vi "BlackJack.vi"() -> ()   [LabVIEW 2018]
panel:
  in  "Description":bool
  in  "Deal cards":bool
  in  "End the game":bool
  out "Dealer's Card":u16[](array[ring])
  out "Your Card":u16[](array[ring])
  out "Result":string
  in  "Number of decks":i32=1
  in  "Chips in hand":dbl=10.0
  in  "Bet":dbl=1.0
  in  "Blackjack odds":dbl=1.5
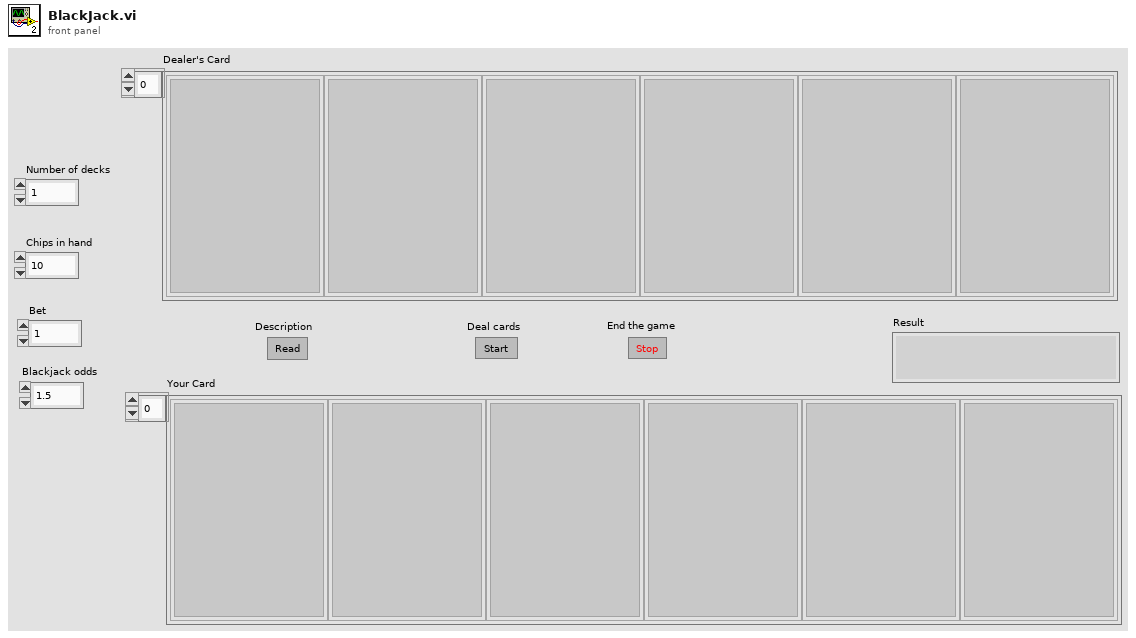
[diagram p1: front panel]
types:
  T1 = enum16{"Left Button", "Center Button", "Right Button", "Window Close"}
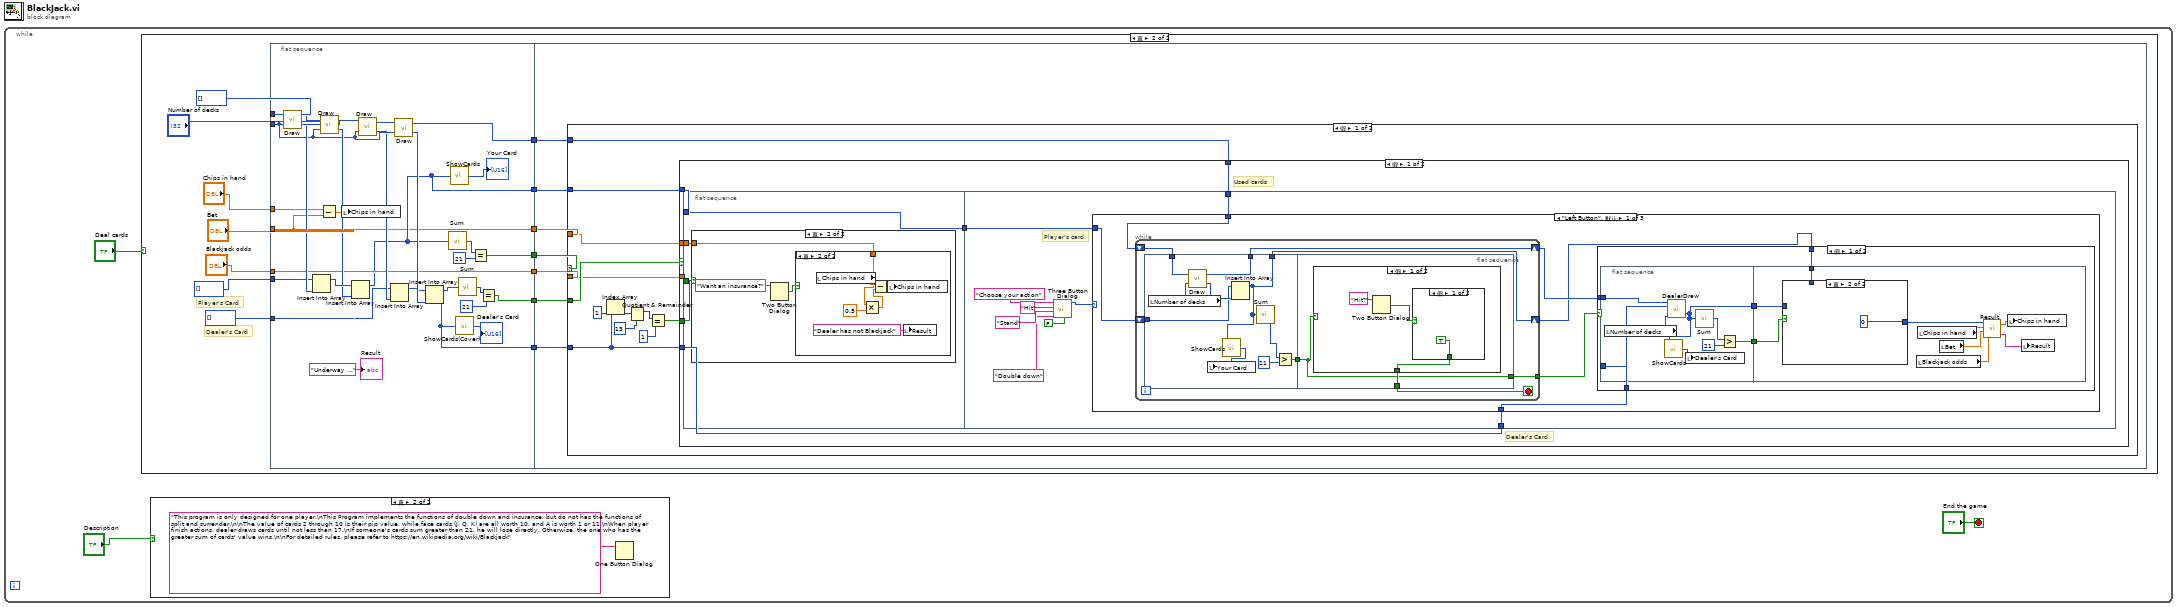
[diagram p0: block diagram]
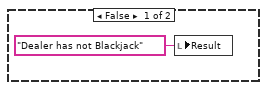
[diagram p5: hidden frame]
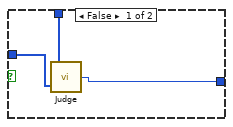
[diagram p6: hidden frame]
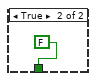
[diagram p8: hidden frame]
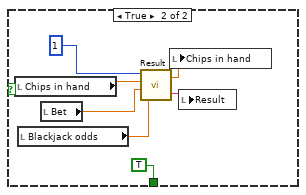
[diagram p9: hidden frame]
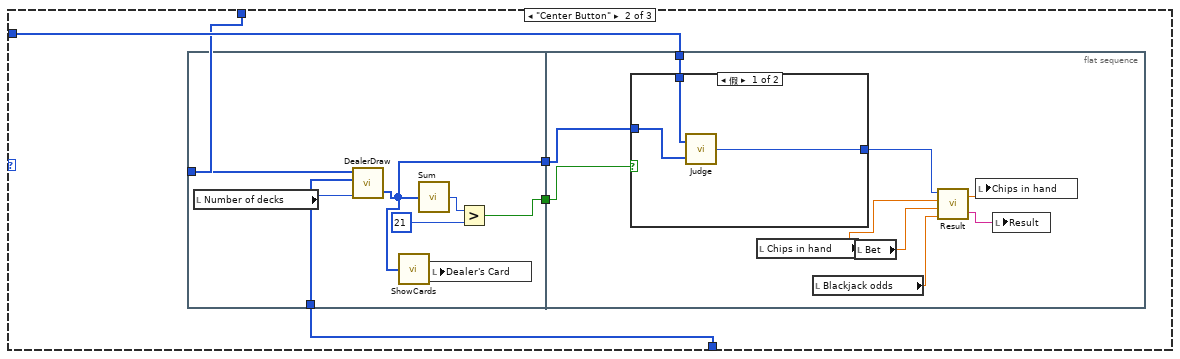
[diagram p10: hidden frame]
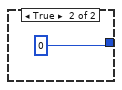
[diagram p11: hidden frame]
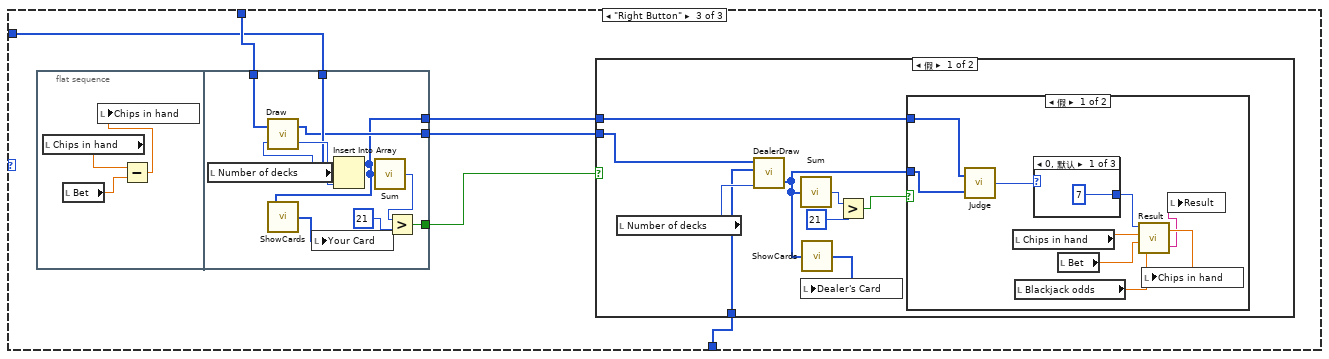
[diagram p12: hidden frame]
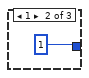
[diagram p13: hidden frame]
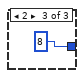
[diagram p14: hidden frame]
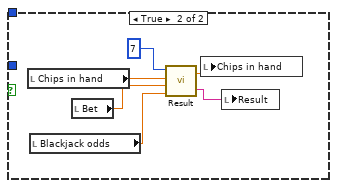
[diagram p15: hidden frame]
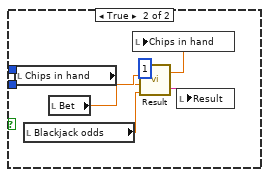
[diagram p16: hidden frame]
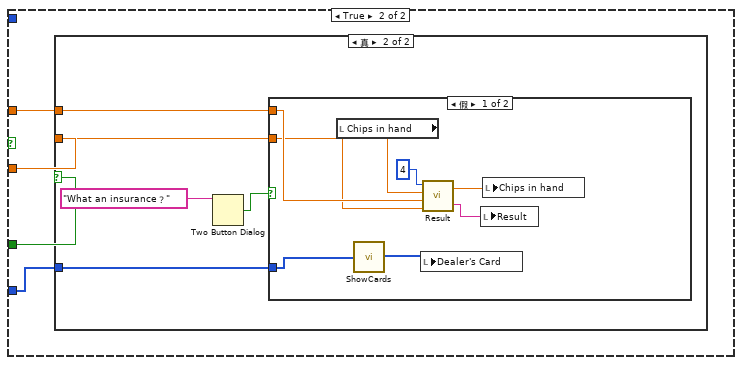
[diagram p17: hidden frame]
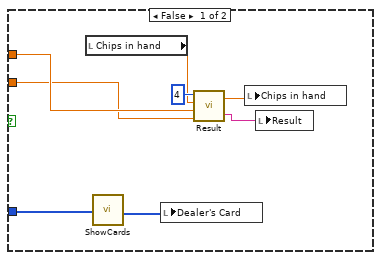
[diagram p18: hidden frame]
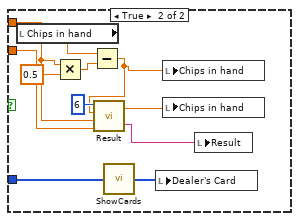
[diagram p19: hidden frame]
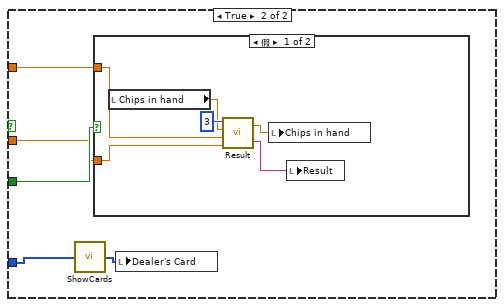
[diagram p20: hidden frame]
diagram:
  n1 = while {
    stop <- "End the game" stop-if-true
    n2 = case shown="真" "Deal cards" {
      frame False {
      }
      frame True {
        # "Player's Card"
        # "Dealer's Card"
        n3 = flat-sequence {
          tunnel: i32[] [] ("输入已用牌") -> [w47]
          tunnel: "Number of decks" -> [w39]
          tunnel: i32[] [] ("数组") -> [w45]
          tunnel: i32[] [] ("数组") -> [w36]
          tunnel: "Bet" -> [w21]
          tunnel: "Blackjack odds" -> [w29]
          tunnel: [w21] -> w18
          tunnel: [w29] -> w17
          tunnel: [w28] -> w16
          tunnel: [w27] -> w15
          tunnel: [w26] -> w14
          tunnel: [w25] -> w13
          tunnel: [w24] -> w12
          tunnel: "Chips in hand" -> [w20]
          tunnel: w18 -> [w54]
          tunnel: w17 -> [w53]
          tunnel: w16 -> [w52]
          tunnel: w15 -> [w51]
          tunnel: w14 -> [w50]
          tunnel: w13 -> [w49]
          tunnel: w12 -> [w48]
          frame #0 {
            n4 = call "Draw.vi"("Number of decks"=w39, "Input used cards"=w47) -> ("No. of card"=w46:i32, "Output used cards"=w44:i32[])
            n5 = Insert Into Array(array=w45, new element=w46) -> (w43:i32[])  [unwired: 1 in]
            n6 = call "Draw.vi"("Number of decks"=w39, "Input used cards"=w44) -> ("No. of card"=w42:i32, "Output used cards"=w41:i32[])
            n7 = Subtract(x=w20, y=w21) -> (x-y=w19:dbl)
            n8 = local write "Chips in hand"(w19) -> ()
            n9 = Insert Into Array(array=w43, new element=w42) -> (w24:i32[])  [unwired: 1 in]
            n10 = call "Draw.vi"("Number of decks"=w39, "Input used cards"=w41) -> ("No. of card"=w38:i32, "Output used cards"=w40:i32[])
            n11 = Insert Into Array(array=w36, new element=w38) -> (w35:i32[])  [unwired: 1 in]
            n12 = call "Draw.vi"("Number of decks"=w39, "Input used cards"=w40) -> ("No. of card"=w37:i32, "Output used cards"=w25:i32[])
            n13 = Insert Into Array(array=w35, new element=w37) -> (w26:i32[])  [unwired: 1 in]
            n14 = call "Sum.vi"("Array"=w24) -> ("Value"=w34:i32)
            n15 = call "ShowCards.vi"("Array 2"=w24) -> ("Array"=→"Your Card":u16[])
            n16 = call "ShowCards(Cover).vi"("Array"=w26) -> ("Array 2"=→"Dealer's Card":u16[])
            n17 = call "Sum.vi"("Array"=w26) -> ("Value"=w32:i32)
            n18 = Equal?(x=w34, y=21) -> (x = y?=w28:bool)
            n19 = Equal?(x=w32, y=21) -> (x = y?=w27:bool)
            "Result" <- "Underway ..." ("结果")
          }
          frame #1 {
            n20 = case shown="假" w52 {
              tunnel: w51 -> [w61 w276]
              tunnel: w54 -> [w59 w275]
              tunnel: w53 -> [w58 w274]
              tunnel: w50 -> [w66 w273]
              tunnel: w49 -> [w57 _]
              tunnel: w48 -> [w56 _]
              frame False {
                n21 = Index Array(array=w66, index=1 ("索引")) -> (element=w65:i32)
                n22 = Quotient & Remainder(x=w65, y=13) -> (x-y*floor(x/y)=w55:i32)  [unwired: 1 out]
                n23 = Equal?(x=w55, y=1) -> (x = y?=w60:bool)
                n24 = case shown="假" w61 {
                  tunnel: w66 -> [w67 w236]
                  tunnel: w60 -> [w72 w239]
                  tunnel: w59 -> [w71 w238]
                  tunnel: w58 -> [_ w237]
                  tunnel: w57 -> [w70 _]
                  tunnel: w56 -> [w68 _]
                  frame False {
                    # "Dealer's Card"
                    # "Used cards"
                    n25 = flat-sequence {
                      tunnel: w72 -> [w75]
                      tunnel: w71 -> [w74]
                      tunnel: [w73] -> w69
                      tunnel: w68 -> [w73]
                      tunnel: w70 -> [w88]
                      tunnel: w69 -> [w87]
                      tunnel: w67 -> [w86]
                      frame #0 {
                        n26 = case shown="真" w75 {
                          tunnel: w74 -> [_ w76]
                          frame False {
                          }
                          frame True {
                            n27 = Two Button Dialog(message="Want an insurance?" ("消息")) -> (T button?=w77:bool)  [unwired: 2 in]
                            n28 = case shown="真" w77 {
                              tunnel: w76 -> [_ w83]
                              frame False {
                                n29 = local write "Result"("Dealer has not Blackjack" ("结果")) -> ()
                              }
                              frame True {
                                n30 = local read "Chips in hand"() -> (w85:dbl)
                                n31 = Multiply(x=w83, y=0.5) -> (x*y=w81:dbl)
                                n32 = Subtract(x=w85, y=w81) -> (x-y=w82:dbl)
                                n33 = local write "Chips in hand"(w82) -> ()
                                n34 = local write "Result"("Dealer has not Blackjack" ("结果")) -> ()
                              }
                            }
                          }
                        }
                      }
                      frame #1 {
                        # "Player's card"
                        n35 = call <vilib>:"Three Button Dialog.vi"("Allow user to close window? (TRUE)"=FALSE, "Right Button Text (\"Cancel\")"="Double down" ("Right Button Text (\"Cancel\")"), "Center Button Text (\"No\")"="Stand" ("Center Button Text (\"No\")"), "Left Button Text (\"Yes\")"="Hit" ("Left Button Text (\"Yes\")"), "message"="Choose your action") -> ("Which Button?"=w89:T1)  [unwired: 6 in]
                        n36 = case shown="\"Left Button\", 默认" w89 {
                          tunnel: w88 -> [w100 w158 w189]
                          tunnel: w87 -> [w97 w159 w188]
                          tunnel: w86 -> [w98 w162 w185]
                          frame "Left Button", Default {
                            n37 = while {
                              tunnel: [w130] -> w99
                              shift-right: [w129] -> w96
                              shift-left: w100 -> [w133]
                              shift-right: [w127] -> w95
                              shift-left: w97 -> [w128]
                              stop <- w131 stop-if-true
                              n38 = flat-sequence {
                                tunnel: w133 -> [w138]
                                tunnel: [w137] -> w132
                                tunnel: [w136] -> w129
                                tunnel: [w135] -> w127
                                tunnel: w128 -> [w134]
                                tunnel: w132 -> [w144]
                                tunnel: [w145] -> w131
                                tunnel: [w144] -> w130
                                frame #0 {
                                n39 = local read "Number of decks"() -> (w139:i32)
                                n40 = call "Draw.vi"("Number of decks"=w139, "Input used cards"=w138) -> ("No. of card"=w143:i32, "Output used cards"=w136:i32[])
                                n41 = Insert Into Array(array=w134, new element=w143) -> (w135:i32[])  [unwired: 1 in]
                                n42 = call "ShowCards.vi"("Array 2"=w135) -> ("Array"=w141:u16[])
                                n43 = local write "Your Card"(w141) -> ()
                                n44 = call "Sum.vi"("Array"=w135) -> ("Value"=w142:i32)
                                n45 = Greater?(x=w142, y=21) -> (0:w137:bool)
                                }
                                frame #1 {
                                n46 = case shown="假" w144 {
                                tunnel: [w146 TRUE] -> w145
                                frame False {
                                n47 = Two Button Dialog(message="Hit?" ("消息")) -> (T button?=w147:bool)  [unwired: 2 in]
                                n48 = case shown="假" w147 {
                                tunnel: [TRUE FALSE] -> w146
                                frame False {
                                }
                                frame True {
                                }
                                }
                                }
                                frame True {
                                n49 = local read "Chips in hand"() -> (w155:dbl)
                                n50 = local read "Blackjack odds"() -> (w153:dbl)
                                n51 = local read "Bet"() -> (w154:dbl)
                                n52 = call "Result.vi"("Blackjack odds"=w153, "Bet"=w154, "Chips before"=w155, "Result"=i16 1 ("结果")) -> ("String"=w152:string, "Chips now"=w151:dbl)
                                n53 = local write "Chips in hand"(w151) -> ()
                                n54 = local write "Result"(w152) -> ()
                                }
                                }
                                }
                              }
                            }
                            n55 = case shown="假" w99 {
                              tunnel: w96 -> [w105 _]
                              tunnel: w98 -> [w104 _]
                              tunnel: w95 -> [w101 _]
                              frame False {
                                n56 = flat-sequence {
                                tunnel: w105 -> [w113]
                                tunnel: w104 -> [w112]
                                tunnel: [w107] -> w103
                                tunnel: [w106] -> w102
                                tunnel: w103 -> [w122]
                                tunnel: w102 -> [w121]
                                tunnel: w101 -> [w120]
                                frame #0 {
                                n57 = local read "Number of decks"() -> (w111:i32)
                                n58 = call "DealerDraw.vi"("Number of decks"=w111, "Input dealer's cards"=w112, "Input used cards"=w113) -> ("Output dealer's cards"=w106:i32[])  [unwired: 1 in, 1 out]
                                n59 = call "ShowCards.vi"("Array 2"=w106) -> ("Array"=w108:u16[])
                                n60 = local write "Dealer's Card"(w108) -> ()
                                n61 = call "Sum.vi"("Array"=w106) -> ("Value"=w110:i32)
                                n62 = Greater?(x=w110, y=21) -> (0:w107:bool)
                                }
                                frame #1 {
                                n63 = case shown="真" w122 {
                                tunnel: w121 -> [w125 _]
                                tunnel: w120 -> [w124 _]
                                tunnel: [w123 0] -> w119
                                frame False {
                                n64 = call "Judge.vi"("Dealer's card"=w125, "Player's card"=w124) -> ("Output result"=w123:i32)
                                }
                                frame True {
                                }
                                }
                                n65 = local read "Blackjack odds"() -> (w114:dbl)
                                n66 = local read "Chips in hand"() -> (w116:dbl)
                                n67 = local read "Bet"() -> (w115:dbl)
                                n68 = call "Result.vi"("Blackjack odds"=w114, "Bet"=w115, "Chips before"=w116, "Result"=w119) -> ("String"=w118:string, "Chips now"=w117:dbl)
                                n69 = local write "Chips in hand"(w117) -> ()
                                n70 = local write "Result"(w118) -> ()
                                }
                                }
                              }
                              frame True {
                              }
                            }
                          }
                          frame "Center Button" {
                            n71 = flat-sequence {
                              tunnel: w158 -> [w169]
                              tunnel: w162 -> [w168]
                              tunnel: [w165] -> w161
                              tunnel: [w164] -> w160
                              tunnel: w161 -> [w173]
                              tunnel: w160 -> [w172]
                              tunnel: w159 -> [w171]
                              frame #0 {
                                n72 = local read "Number of decks"() -> (w170:i32)
                                n73 = call "DealerDraw.vi"("Number of decks"=w170, "Input dealer's cards"=w168, "Input used cards"=w169) -> ("Output dealer's cards"=w164:i32[])  [unwired: 1 in, 1 out]
                                n74 = call "ShowCards.vi"("Array 2"=w164) -> ("Array"=w163:u16[])
                                n75 = call "Sum.vi"("Array"=w164) -> ("Value"=w167:i32)
                                n76 = local write "Dealer's Card"(w163) -> ()
                                n77 = Greater?(x=w167, y=21) -> (0:w165:bool)
                              }
                              frame #1 {
                                n78 = case shown="假" w173 {
                                tunnel: w171 -> [w182 _]
                                tunnel: w172 -> [w181 _]
                                tunnel: [w180 0] -> w174
                                frame False {
                                n79 = call "Judge.vi"("Dealer's card"=w181, "Player's card"=w182) -> ("Output result"=w180:i32)
                                }
                                frame True {
                                }
                                }
                                n80 = local read "Chips in hand"() -> (w177:dbl)
                                n81 = local read "Blackjack odds"() -> (w175:dbl)
                                n82 = local read "Bet"() -> (w176:dbl)
                                n83 = call "Result.vi"("Blackjack odds"=w175, "Bet"=w176, "Chips before"=w177, "Result"=w174) -> ("String"=w179:string, "Chips now"=w178:dbl)
                                n84 = local write "Chips in hand"(w178) -> ()
                                n85 = local write "Result"(w179) -> ()
                              }
                            }
                          }
                          frame "Right Button" {
                            n86 = flat-sequence {
                              tunnel: w189 -> [w235]
                              tunnel: w188 -> [w232]
                              tunnel: [w229] -> w187
                              tunnel: [w228] -> w186
                              tunnel: [w227] -> w184
                              frame #0 {
                                n87 = local read "Chips in hand"() -> (w224:dbl)
                                n88 = local read "Bet"() -> (w225:dbl)
                                n89 = Subtract(x=w224, y=w225) -> (x-y=w223:dbl)
                                n90 = local write "Chips in hand"(w223) -> ()
                              }
                              frame #1 {
                                n91 = local read "Number of decks"() -> (w234:i32)
                                n92 = call "Draw.vi"("Number of decks"=w234, "Input used cards"=w235) -> ("No. of card"=w233:i32, "Output used cards"=w228:i32[])
                                n93 = Insert Into Array(array=w232, new element=w233) -> (w227:i32[])  [unwired: 1 in]
                                n94 = call "ShowCards.vi"("Array 2"=w227) -> ("Array"=w226:u16[])
                                n95 = local write "Your Card"(w226) -> ()
                                n96 = call "Sum.vi"("Array"=w227) -> ("Value"=w231:i32)
                                n97 = Greater?(x=w231, y=21) -> (0:w229:bool)
                              }
                            }
                            n98 = case shown="假" w187 {
                              tunnel: w186 -> [w196 _]
                              tunnel: w185 -> [w197 _]
                              tunnel: w184 -> [w192 _]
                              frame False {
                                n99 = local read "Number of decks"() -> (w198:i32)
                                n100 = call "DealerDraw.vi"("Number of decks"=w198, "Input dealer's cards"=w197, "Input used cards"=w196) -> ("Output dealer's cards"=w191:i32[])  [unwired: 1 in, 1 out]
                                n101 = call "Sum.vi"("Array"=w191) -> ("Value"=w195:i32)
                                n102 = call "ShowCards.vi"("Array 2"=w191) -> ("Array"=w190:u16[])
                                n103 = local write "Dealer's Card"(w190) -> ()
                                n104 = Greater?(x=w195, y=21) -> (0:w193:bool)
                                n105 = case shown="假" w193 {
                                tunnel: w192 -> [w207 _]
                                tunnel: w191 -> [w206 _]
                                frame False {
                                n106 = call "Judge.vi"("Dealer's card"=w206, "Player's card"=w207) -> ("Output result"=w205:i32)
                                n107 = local read "Chips in hand"() -> (w202:dbl)
                                n108 = local read "Blackjack odds"() -> (w200:dbl)
                                n109 = case shown="0, 默认" w205 {
                                tunnel: [7 1 8] -> w204
                                frame 0, Default {
                                }
                                frame 1 {
                                }
                                frame 2 {
                                }
                                }
                                n110 = local read "Bet"() -> (w201:dbl)
                                n111 = call "Result.vi"("Blackjack odds"=w200, "Bet"=w201, "Chips before"=w202, "Result"=w204) -> ("String"=w199:string, "Chips now"=w203:dbl)
                                n112 = local write "Chips in hand"(w203) -> ()
                                n113 = local write "Result"(w199) -> ()
                                }
                                frame True {
                                n114 = local read "Chips in hand"() -> (w215:dbl)
                                n115 = local read "Blackjack odds"() -> (w212:dbl)
                                n116 = local read "Bet"() -> (w213:dbl)
                                n117 = call "Result.vi"("Blackjack odds"=w212, "Bet"=w213, "Chips before"=w215, "Result"=i16 7 ("结果")) -> ("String"=w211:string, "Chips now"=w214:dbl)
                                n118 = local write "Chips in hand"(w214) -> ()
                                n119 = local write "Result"(w211) -> ()
                                }
                                }
                              }
                              frame True {
                                n120 = local read "Chips in hand"() -> (w221:dbl)
                                n121 = local read "Blackjack odds"() -> (w219:dbl)
                                n122 = local read "Bet"() -> (w220:dbl)
                                n123 = call "Result.vi"("Blackjack odds"=w219, "Bet"=w220, "Chips before"=w221, "Result"=i16 1 ("结果")) -> ("String"=w217:string, "Chips now"=w218:dbl)
                                n124 = local write "Chips in hand"(w218) -> ()
                                n125 = local write "Result"(w217) -> ()
                              }
                            }
                          }
                        }
                      }
                    }
                  }
                  frame True {
                    n126 = case shown="真" w239 {
                      tunnel: w238 -> [w246 w250]
                      tunnel: w237 -> [w245 w249]
                      tunnel: w236 -> [w241 w248]
                      frame False {
                        n127 = local read "Chips in hand"() -> (w242:dbl)
                        n128 = call "ShowCards.vi"("Array 2"=w241) -> ("Array"=w240:u16[])
                        n129 = local write "Dealer's Card"(w240) -> ()
                        n130 = call "Result.vi"("Blackjack odds"=w245, "Bet"=w246, "Chips before"=w242, "Result"=i16 4 ("结果")) -> ("String"=w243:string, "Chips now"=w244:dbl)
                        n131 = local write "Chips in hand"(w244) -> ()
                        n132 = local write "Result"(w243) -> ()
                      }
                      frame True {
                        n133 = Two Button Dialog(message="What an insurance？" ("消息")) -> (T button?=w251:bool)  [unwired: 2 in]
                        n134 = case shown="假" w251 {
                          tunnel: w250 -> [w259 w267]
                          tunnel: w249 -> [w258 w270]
                          tunnel: w248 -> [w255 w263]
                          frame False {
                            n135 = local read "Chips in hand"() -> (w253:dbl)
                            n136 = call "ShowCards.vi"("Array 2"=w255) -> ("Array"=w254:u16[])
                            n137 = local write "Dealer's Card"(w254) -> ()
                            n138 = call "Result.vi"("Blackjack odds"=w258, "Bet"=w259, "Chips before"=w253, "Result"=i16 4 ("结果")) -> ("String"=w256:string, "Chips now"=w257:dbl)
                            n139 = local write "Result"(w256) -> ()
                            n140 = local write "Chips in hand"(w257) -> ()
                          }
                          frame True {
                            n141 = local read "Chips in hand"() -> (w261:dbl)
                            n142 = Multiply(x=w267, y=0.5) -> (x*y=w265:dbl)
                            n143 = Subtract(x=w261, y=w265) -> (x-y=w264:dbl)
                            n144 = call "Result.vi"("Blackjack odds"=w270, "Bet"=w267, "Chips before"=w264, "Result"=i16 6 ("结果")) -> ("String"=w268:string, "Chips now"=w269:dbl)
                            n145 = call "ShowCards.vi"("Array 2"=w263) -> ("Array"=w262:u16[])
                            n146 = local write "Dealer's Card"(w262) -> ()
                            n147 = local write "Chips in hand"(w264) -> ()
                            n148 = local write "Chips in hand"(w269) -> ()
                            n149 = local write "Result"(w268) -> ()
                          }
                        }
                      }
                    }
                  }
                }
              }
              frame True {
                n150 = call "ShowCards.vi"("Array 2"=w273) -> ("Array"=w272:u16[])
                n151 = case shown="假" w276 {
                  tunnel: w275 -> [w282 w288]
                  tunnel: w274 -> [w281 w287]
                  frame False {
                    n152 = local read "Chips in hand"() -> (w277:dbl)
                    n153 = call "Result.vi"("Blackjack odds"=w281, "Bet"=w282, "Chips before"=w277, "Result"=i16 3 ("结果")) -> ("String"=w279:string, "Chips now"=w280:dbl)
                    n154 = local write "Chips in hand"(w280) -> ()
                    n155 = local write "Result"(w279) -> ()
                  }
                  frame True {
                    n156 = local read "Chips in hand"() -> (w283:dbl)
                    n157 = call "Result.vi"("Blackjack odds"=w287, "Bet"=w288, "Chips before"=w283, "Result"=i16 5 ("结果")) -> ("String"=w284:string, "Chips now"=w285:dbl)
                    n158 = local write "Result"(w284) -> ()
                    n159 = local write "Chips in hand"(w285) -> ()
                  }
                }
                n160 = local write "Dealer's Card"(w272) -> ()
              }
            }
          }
        }
      }
    }
    n161 = case shown="真" "Description" {
      frame False {
      }
      frame True {
        n162 = One Button Dialog(message="This program is only designed for one player.\nThis Program implements the functions of double down and insurance, but do not has the functions of split and surrender.\n\nThe value of cards 2 through 10 is their pip value, while face cards (J, Q, K) are all worth 10, and A is worth 1 or 11.\nWhen player finish actions, dealer draws cards until not less than 17.\nIf someone's cards sum greater than 21, he will lose directly. Otherwise, the one who has the greater sum of cards' value wins.\n\nFor detailed rules, please refer to https://en.wikipedia.org/wiki/Blackjack" ("消息")) -> ()  [unwired: 1 in, 1 out]
      }
    }
  }
